vi "Revision Query.vi"(8 "error in (no error)":errorcluster) -> (0 "error out":errorcluster, 2 "Instrument Driver Revision":string)   [LabVIEW 2018, in "Agilent 87XX Series.lvlib"]
uses:
  Agilent 87XX Series.lvlib
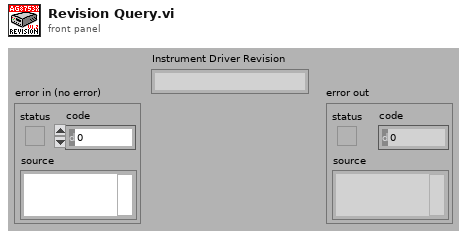
[diagram p1: front panel]
types:
  T1 = enum32{"invalid app kind", "Development System", "Run Time System", "Student Edition", "Embedded LabVIEW", "Evaluation", "Custom"}
  T2 = cluster{"Major":u16, "Minor":u16, "Fix":u16, "Build":u16}
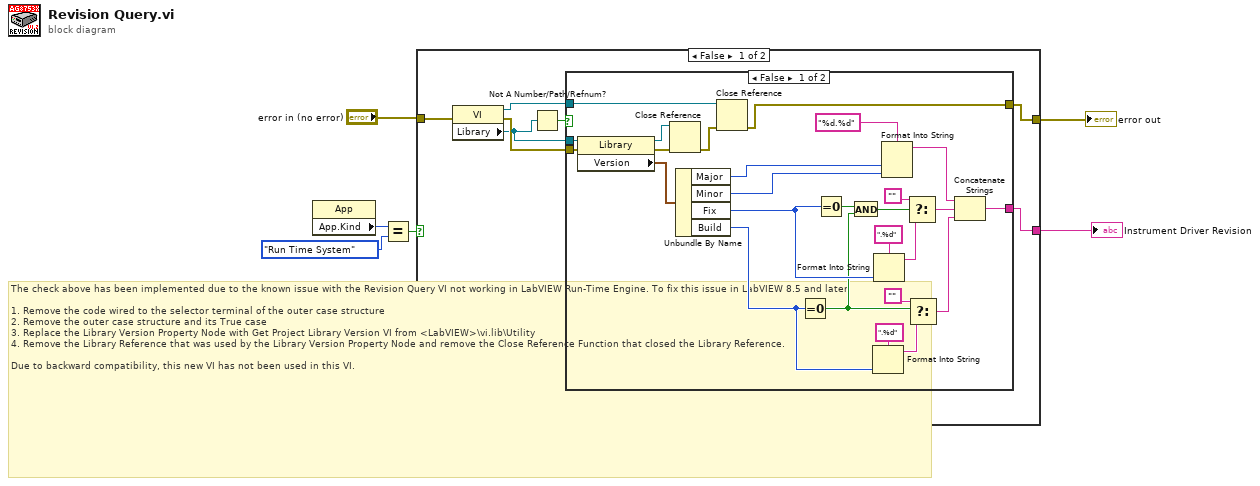
[diagram p0: block diagram]
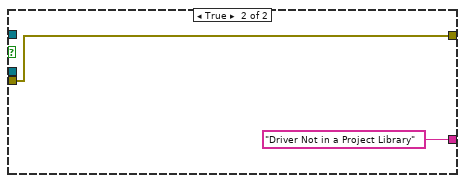
[diagram p2: hidden frame]
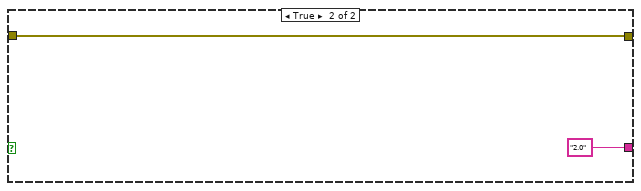
[diagram p3: hidden frame]
diagram:
  # "The check above has been implemented due to the known issue with the Revision Query VI not working in LabVIEW Run-Time Engine. To fix this issue in LabVIEW 8.5 and later:\n\n1. Remove the code wired to the selector terminal of the outer case structure\n2. Remove the outer case structure and its True case\n3. Replace the Library Version Property Node with Get Project Library Version VI from <LabVIEW>\\vi.lib\\Utility\n4. Remove the Library Reference that was used by the Library Version Property Node and remove the Close Reference Function that closed the Library Reference.\n\nDue to backward compatibility, this new VI has not been used in this VI."
  n1 = property class="App"() -> ("App.Kind"=w5:T1)  [unwired: 2 in, 2 out]
  n2 = Equal?(x=w5, y=T1."Run Time System") -> (x = y?=w6:bool)
  n3 = case shown="False" w6 {
    tunnel: "error in (no error)" -> [w13 w43]
    tunnel: [w8 "2.0"] -> w1
    tunnel: [w7 w43] -> w2
    frame False {
      n4 = property class="VI"(error in=w13) -> (reference out=w9:refnum<vi>, error out=w12:errorcluster, "Library"=w11:refnum<vi>)  [unwired: 1 in]
      n5 = Not A Number/Path/Refnum?(number/path/refnum=w11) -> (NaN/Path/Refnum?=w10:bool)
      n6 = case shown="False" w10 {
        tunnel: [w18 w40] -> w7
        tunnel: [w17 "Driver Not in a Project Library"] -> w8
        tunnel: w12 -> [w16 w40]
        tunnel: w11 -> [w15 _]
        tunnel: w9 -> [w14 _]
        frame False {
          n7 = property class="Library"(reference=w15, error in=w16) -> (reference out=w38:refnum<vi>, error out=w39:errorcluster, "Version"=w36:T2)
          n8 = Close Reference(reference=w38, error in (no error)=w39) -> (error out=w37:errorcluster)
          n9 = Unbundle By Name(w36) -> ("Major"=w25:u16, "Minor"=w24:u16, "Fix"=w22:u16, "Build"=w23:u16)
          n10 = Close Reference(reference=w14, error in (no error)=w37) -> (error out=w18:errorcluster)
          n11 = Equal To 0?(x=w23) -> (x = 0?=w20:bool)
          n12 = Equal To 0?(x=w22) -> (x = 0?=w21:bool)
          n13 = And(x=w21, y=w20) -> (x .and. y?=w19:bool)
          n14 = Format Into String(format string=".%d", w23) -> (resulting string=w29:string)  [unwired: 2 in, 1 out]
          n15 = Format Into String(format string=".%d", w22) -> (resulting string=w33:string)  [unwired: 2 in, 1 out]
          n16 = Format Into String(format string="%d.%d", w25, w24) -> (resulting string=w31:string)  [unwired: 2 in, 1 out]
          n17 = Select(t="", s=w19, f=w33) -> (s? t:f=w30:string)
          n18 = Select(t="", s=w20, f=w29) -> (s? t:f=w26:string)
          n19 = Concatenate Strings(w31, w30, w26) -> (w17:string)
        }
        frame True {
        }
      }
    }
    frame True {
    }
  }
  "Instrument Driver Revision" <- w1
  "error out" <- w2
